vi "Replace Missing Items In Hierarchy.vi"(11 "Flat Hierarchy":T1) -> (3 "Flat Hierarchy":T1)   [LabVIEW 2014, in "PL Framework Configuration Tool.lvlib" / "SystemConfigRepo.lvclass"]
doc: "Replace classes in Flat Hierarchy with \"Missing Plugin configuration.lvclass\" if they are not found in memory or by the class discovery singleton."
uses:
  SystemConfigRepo.lvclass
  <vilib>/NI/Configuration Framework/tree serializer/flat hierarchy.ctl
  <vilib>/NI/Configuration Framework/tree serializer/full hierarchy.ctl
  <vilib>/NI/Configuration Framework/tree serializer/hierarchy element.ctl
  <vilib>/NI/Configuration Framework/tree serializer/instance data.ctl
  <vilib>/NI/Configuration Framework/class discovery singleton/class discovery singleton methods.ctl
  <vilib>/NI/Configuration Framework/class discovery singleton/class discovery singleton.lvlib
  <vilib>/NI/Configuration Framework/tree serializer/NISE_CEF_TreeSerializer.lvlib
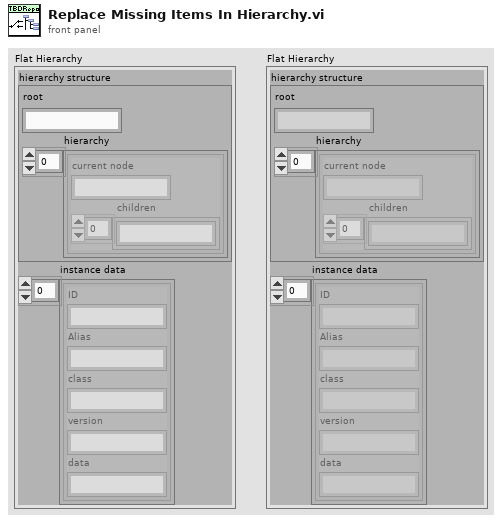
[diagram p1: front panel]
types:
  T1 = typedef "NISE_CEF_TreeSerializer.lvlib/flat hierarchy.ctl" = cluster{"hierarchy structure":T2, "instance data":T4[]}
  T2 = typedef "NISE_CEF_TreeSerializer.lvlib/full hierarchy.ctl" = cluster{"root":string, "hierarchy":T3[]}
  T3 = typedef "NISE_CEF_TreeSerializer.lvlib/hierarchy element.ctl" = cluster{"current node":string, "children":string[]}
  T4 = typedef "NISE_CEF_TreeSerializer.lvlib/instance data.ctl" = cluster{"ID":string, "Alias":string, "class":string, "version":string, "data":string}
  T5 = typedef "class discovery singleton.lvlib/class discovery singleton methods.ctl" = enum16{"add search paths", "load class by name", "list available classes", "get class path", "delete cache"}
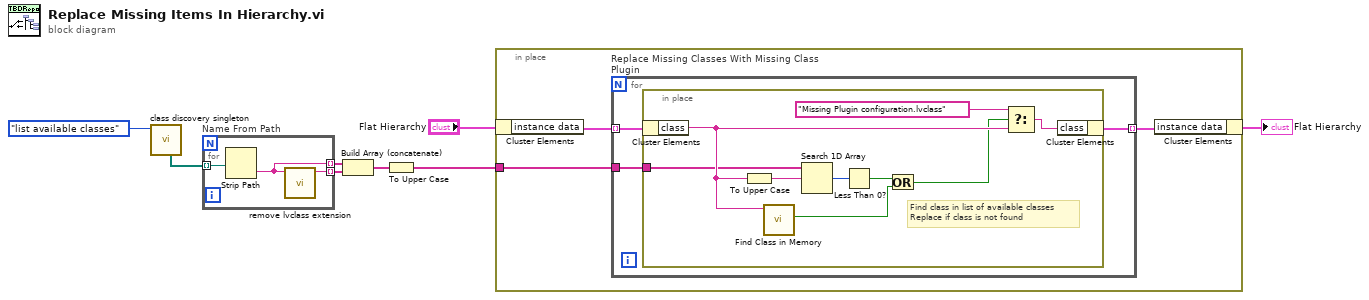
[diagram p0: block diagram]
diagram:
  n1 = call <vilib>:"class discovery singleton.vi"("method"=class_discovery_singleton_methods."list available classes") -> ("discovered classes"=w2:path[])  [unwired: 7 in, 3 out]
  n2 = for "Name From Path" {
    tunnel: w2 -> [w11] mode=indexing
    tunnel: [w10] -> w4 mode=indexing
    tunnel: [w9] -> w3 mode=indexing
    n3 = Strip Path(path=w11) -> (name=w9:string)  [unwired: 1 out]
    n4 = call <vilib>:"remove lvclass extension.vi"("class name in"=w9) -> ("class name out"=w10:string)  [unwired: 10 in]
  }
  n5 = Build Array (concatenate)(w3, w4) -> (w5:string[])
  n6 = To Upper Case(1:w5) -> (0:w1:string[])
  n7 = in-place {
    in-place-border: w1 -> [w12]
    n8 = in-place-cluster #1("Flat Hierarchy") -> ("instance data"=w14:T4[])
    n9 = for "Replace Missing Classes With Missing Class Plugin" {
      tunnel: w14 -> [w17] mode=indexing
      tunnel: [w16] -> w13 mode=indexing
      tunnel: w12 -> [w15]
      n10 = in-place {
        in-place-border: w15 -> [w18]
        # "Find class in list of available classes\nReplace if class is not found"
        n11 = in-place-cluster #2(w17) -> ("class"=w22:string)
        n12 = To Upper Case(1:w22) -> (0:w26:string)
        n13 = call "Find Class in Memory.vi"("Class Name"=w22) -> ("Class Found?"=w20:bool)  [unwired: 9 in, 1 out]
        n14 = Search 1D Array(1D array=w18, element=w26) -> (index of element=w25:i32)  [unwired: 1 in]
        n15 = Less Than 0?(x=w25) -> (x < 0?=w21:bool)
        n16 = Or(x=w21, y=w20) -> (x .or. y?=w19:bool)
        n17 = Select(t="Missing Plugin configuration.lvclass", s=w19, f=w22) -> (s? t:f=w24:string)
        n18 = in-place-cluster #2("class"=w24) -> (w16:T4)
      }
    }
    n19 = in-place-cluster #1("instance data"=w13) -> (→"Flat Hierarchy":T1)
  }
